vi "Facade.vi"(0 "Data In":T7, 2 "Display State In":T2, 3 "Container State":T6) -> (6 "Data Out":T7, 7 "Display State Out":T2, 8 "Action":T1)   [LabVIEW 2020, in "FSM Editor.xctl"]
uses:
  FSM Editor.xctl
  <vilib>/_xctls/Action.ctl
  <vilib>/_xctls/XControlSupport.lvlib
  Classes/FSM.Graph/FSM.Graph.lvclass
  <vilib>/Utility/cursorutil.llb/Set Cursor (Icon Pict).vi
  Drag Mode.ctl
  Classes/FSM.Edge/FSM.Edge.lvclass
  <vilib>/_xctls/Container State.ctl
  Data.vi
  State.vi
  <vilib>/Utility/miscctls.llb/LVPoint32TypeDef.ctl
  Classes/FSM.Port/FSM.Port.lvclass
  Events.ctl
  NodeAdded.ctl
  NodeSelected.ctl
  EdgeEventData.ctl
panel:
  out "picture":picture
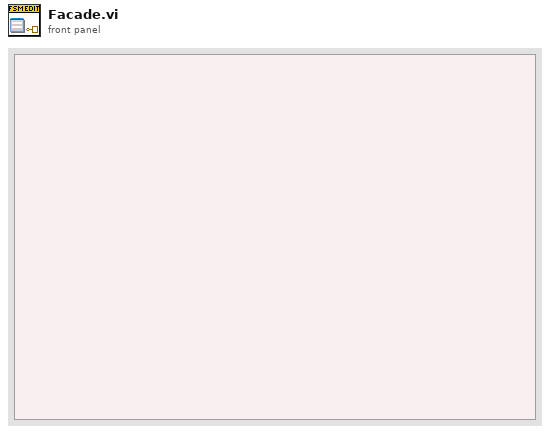
[diagram p1: front panel]
types:
  T1 = typedef "XControlSupport.lvlib/Action.ctl" = cluster{"Data Changed?":bool, "State Changed?":bool, "Action Name":string}
  T2 = typedef "FSM Editor.xctl/State.vi" = cluster{"snap":bool, "default name":string, "dragStartPoint":T3, "dragMode":T4, "gridsize":dbl, "selectRect":cluster{"left":i16, "top":i16, "right":i16, "bottom":i16}, "events":string[], "cs+/cs-":bool, "insertEdgeAt":string, "insertingEdge":bool, "activePort":refnum<class "FSM.Port.lvclass">, "sourcePort":refnum<class "FSM.Port.lvclass">, "insertionEnd":cluster{"x":i16, "y":i16}, "insertEdgeSpec":string, "nodeIndex":i32, "Events":T5, "action":string}
  T3 = typedef "LVPoint32TypeDef.ctl" = cluster{"Horizontal":i32, "Vertical":i32}
  T4 = typedef "Drag Mode.ctl" = enum16{"Off", "NodePending", "Nodes", "Pan", "Select", "EdgeInsertion", "EdgePoint", "EdgeLabel"}
  T5 = typedef "FSM Editor.xctl/Events.ctl" = cluster{"NodeAdded":refnum<user-event>, "NodeSelected":refnum<user-event>, "NodeDeleted":refnum<user-event>, "EdgeAdded":refnum<user-event>, "EdgeDeleted":refnum<user-event>, "EdgeSelected":refnum<user-event>}
  T6 = typedef "XControlSupport.lvlib/Container State.ctl" = cluster{"Indicator?":bool, "Run Mode?":bool, " Refnum":refnum<vi>}
  T7 = typedef "FSM Editor.xctl/Data.vi" = refnum<class "FSM.Graph.lvclass">
  T8 = cluster{"left":i16, "top":i16, "right":i16, "bottom":i16}
  T9 = cluster{"SourceName":string, "TargetName":string, "Accessors:Text":string, "Type":string}
  T10 = cluster{"Shift":bool, "Ctrl":bool, "Alt":bool, "Cmd":bool, "Opt":bool}
  T11 = typedef "LVBoundsTypeDef.ctl" = cluster{"Width":u32, "Height":u32}
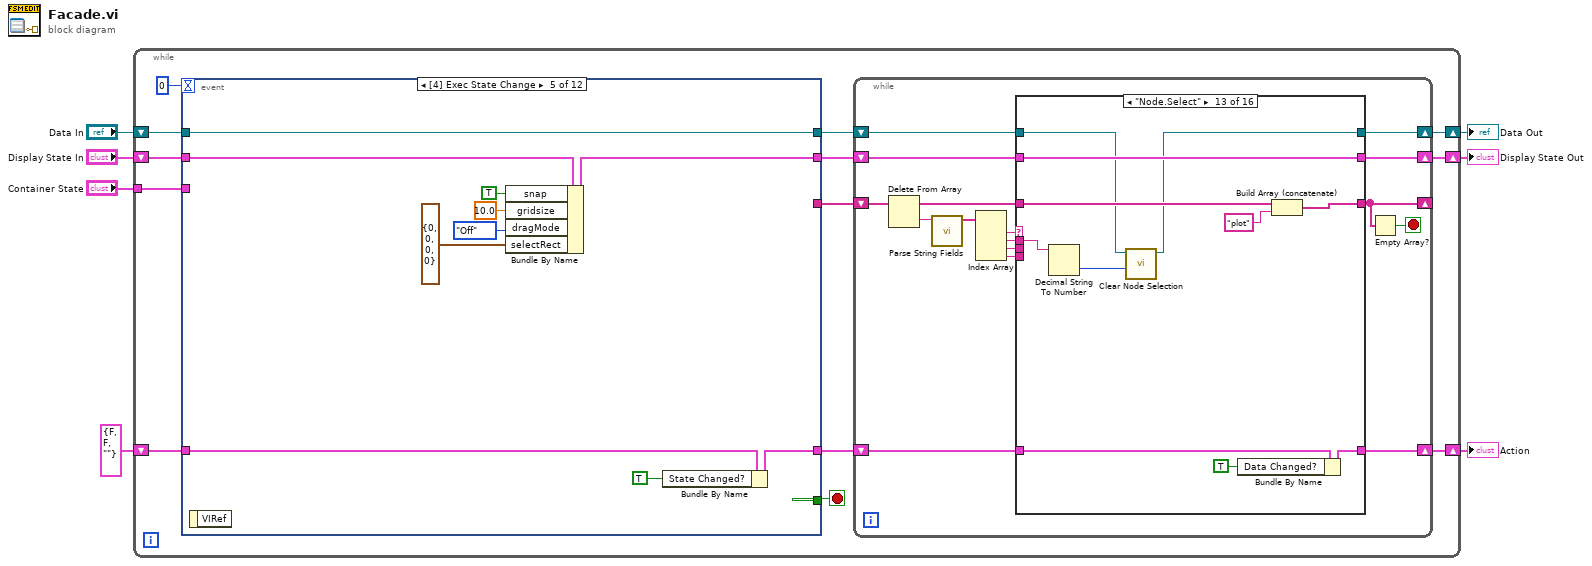
[diagram p0: block diagram]
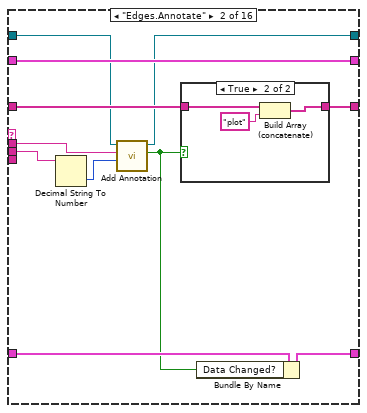
[diagram p3: hidden frame]
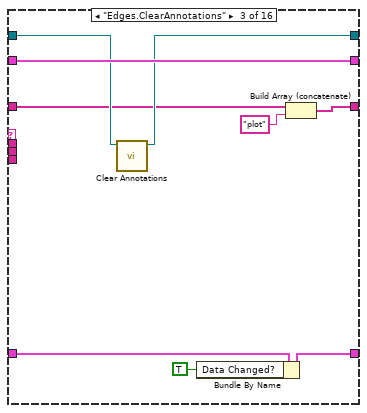
[diagram p5: hidden frame]
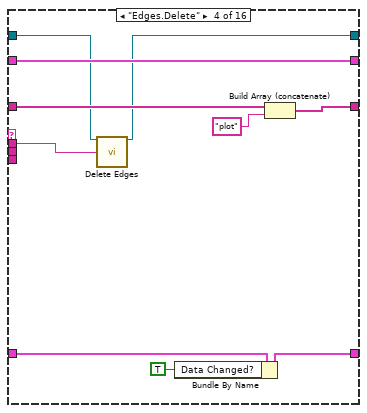
[diagram p6: hidden frame]
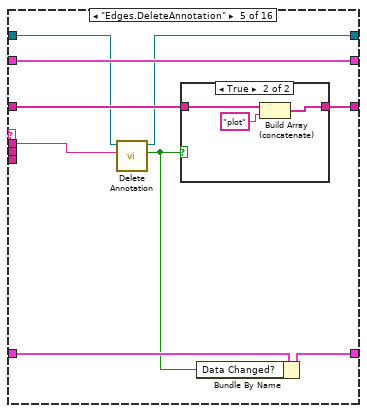
[diagram p7: hidden frame]
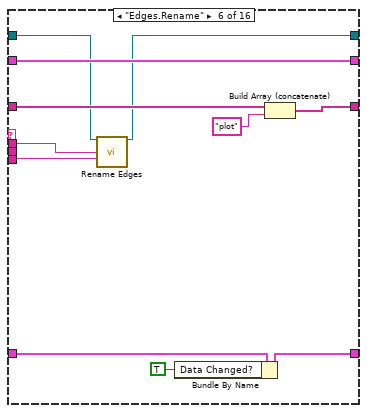
[diagram p9: hidden frame]
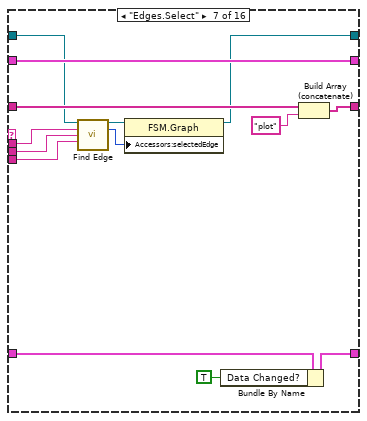
[diagram p10: hidden frame]
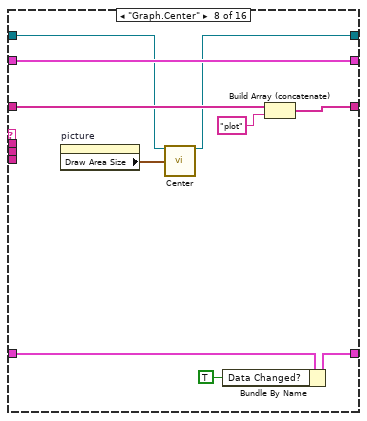
[diagram p11: hidden frame]
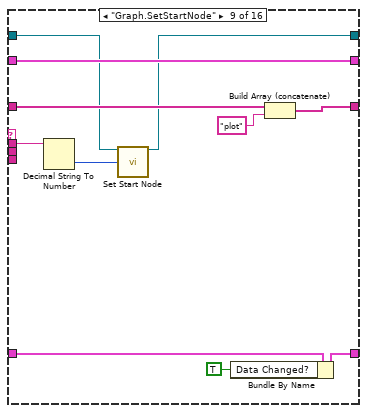
[diagram p12: hidden frame]
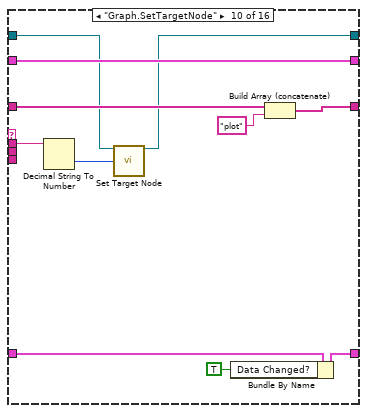
[diagram p13: hidden frame]
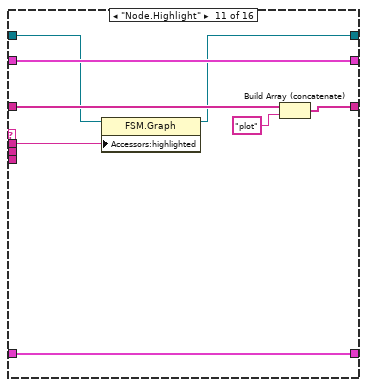
[diagram p14: hidden frame]
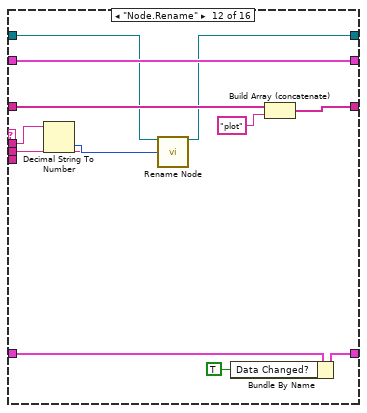
[diagram p15: hidden frame]
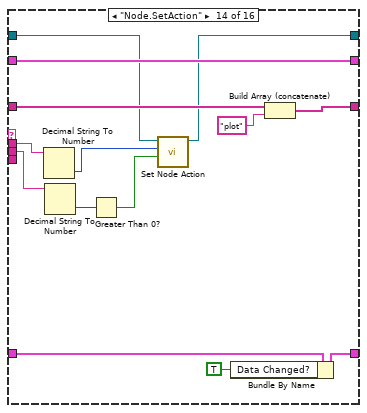
[diagram p16: hidden frame]
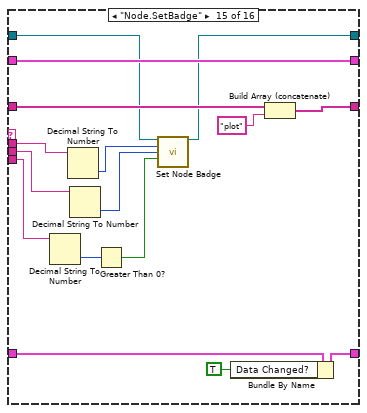
[diagram p17: hidden frame]
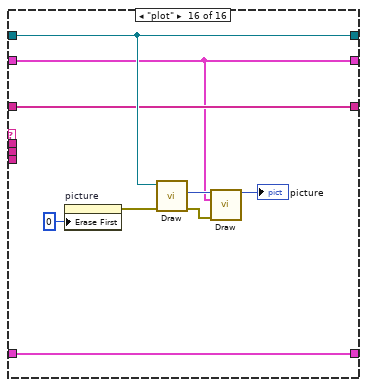
[diagram p18: hidden frame]
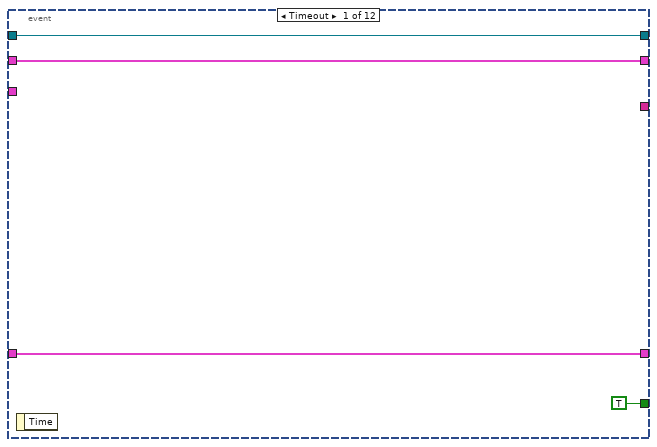
[diagram p19: hidden frame]
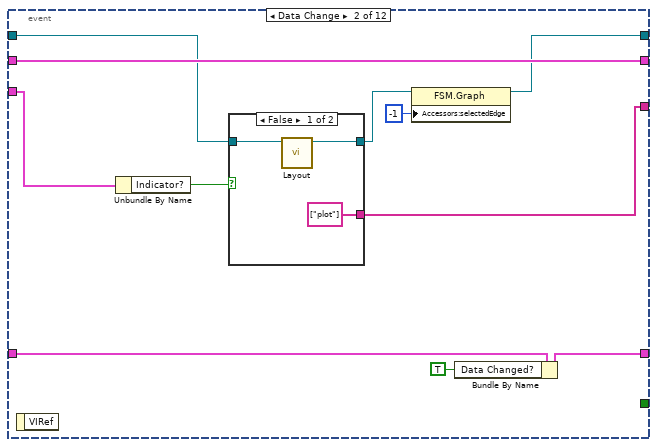
[diagram p20: hidden frame]
diagram:
  n1 = while {
    shift-right: [w10] -> w4
    shift-left: "Display State In" -> [w20]
    tunnel: "Container State" -> [w17]
    shift-right: [w8] -> w7
    shift-left: "Data In" -> [w16]
    shift-right: [w11] -> w2
    shift-left: T1 {"Data Changed?"=FALSE, "State Changed?"=FALSE, "Action Name"=""} ("Action") -> [w15]
    stop <- w19 stop-if-true
    n2 = event shown="[4] Exec State Change" {
      selector: _ -> [_ _ _ _ _ _ _ _ _ _ _ _]
      dyn-events: _ -> [_ _ _ _ _ _ _ _ _ _ _ _]
      timeout: 0 -> [_ _ _ _ _ _ _ _ _ _ _ _]
      tunnel: w20 -> [w216 w229 w241 w246 w256 w269 w273 w295 w362 w383 w399 w425]
      tunnel: [w216 w229 w238 w246 w254 w269 w276 w289 w361 w382 w398 w420] -> w13
      tunnel: [TRUE _ _ _ _ _ _ _ _ _ _ _] -> w19
      tunnel: w17 -> [_ w223 _ _ _ _ w271 w284 w357 _ w389 w416]
      tunnel: w16 -> [w215 w220 w243 w245 w247 w268 w278 w293 w363 w384 w401 w424]
      tunnel: [w215 w226 w243 w245 w247 w268 w277 w292 w364 w385 w400 w424] -> w9
      tunnel: [w217 w225 w236 w244 w253 w267 w275 w291 w358 w380 w391 w422] -> w12
      tunnel: w15 -> [w217 w228 w242 w244 w255 w267 w280 w296 w365 w386 w402 w423]
      tunnel: [_ w221 w239 _ _ _ _ w281 _ w378 w394 string[] ["plot"] ("f")] -> w14
      event Timeout {
        n3 = event-data() -> ()  [unwired: 1 in, 1 out]
      }
      event Data Change {
        n4 = event-data() -> ()  [unwired: 1 in, 1 out]
        n5 = Unbundle By Name(w223) -> ("Indicator?"=w222:bool)
        n6 = case shown="False" w222 {
          tunnel: [string[] ["plot"] string[] ["Graph.Center"]] -> w221
          tunnel: w220 -> [w231 w233]
          tunnel: [w230 w233] -> w219
          frame False {
            n7 = call "Layout.vi"("FSM in"=w231) -> ("FSM out"=w230:T7)  [unwired: 9 in, 1 out]
          }
          frame True {
          }
        }
        n8 = property class="FSM.Graph"(reference=w219, "Accessors:selectedEdge"=-1 ("selectedEdge")) -> (reference out=w226:T7)  [unwired: 1 in, 1 out]
        n9 = Bundle By Name(cluster=w228, "Data Changed?"=TRUE) -> (w225:T1)
      }
      event Display State Change {
        n10 = event-data() -> ()  [unwired: 1 in, 1 out]
        n11 = Unbundle By Name(w241) -> ("action"=w240:string)
        n12 = Bundle By Name(cluster=w242, "State Changed?"=TRUE) -> (w236:T1)
        n13 = Bundle By Name(cluster=w241, "action"="") -> (w238:T2)
        n14 = Build Array(w240) -> (w239:string[])
      }
      event Direction Change {
        n15 = event-data() -> ()  [unwired: 1 in, 1 out]
      }
      event Exec State Change {
        n16 = event-data() -> ()  [unwired: 1 in, 1 out]
        n17 = Bundle By Name(cluster=w256, "snap"=TRUE, "gridsize"=10.0, "dragMode"=Drag_Mode."Off", "selectRect"=T8 {"left"=0, "top"=0, "right"=0, "bottom"=0}) -> (w254:T2)
        n18 = Bundle By Name(cluster=w255, "State Changed?"=TRUE) -> (w253:T1)
      }
      event Panel Resize {
        w260 = i16 10
        n19 = event-data() -> ("NewBnds.Right"=w266:i16, "NewBnds.Left"=w265:i16, "NewBnds.Bottom"=w264:i16, "NewBnds.Top"=w263:i16)  [unwired: 1 in]
        n20 = Subtract(x=w266, y=w265) -> (x-y=w262:i16)
        n21 = Subtract(x=w264, y=w263) -> (x-y=w261:i16)
        n22 = Add(x=w262, y=w260) -> (x+y=w259:i16)
        n23 = Add(x=w261, y=w260) -> (x+y=w258:i16)
        n24 = Bundle(w259, w258) -> (w257:cluster{i16, i16})  [unwired: 1 in]
        n25 = property on="picture" class="Pict"("Draw Area Size"=w257) -> ()  [unwired: 2 in, 2 out]
      }
      event "picture": Shortcut Menu Activation? {
        n26 = event-data() -> ("MenuRef"=w272:refnum<k9>, "Coords"=w279:T3)  [unwired: 1 in]
        n27 = Unbundle By Name(w271) -> ("Indicator?"=w270:bool)
        n28 = call "Build Context Menu.vi"("FSM.Graph in"=w278, "Display State In in"=w273, "MenuRef"=w272, "Coords"=w279) -> ("FSM.Graph out"=w277:T7, "Display State In out"=w276:T2)  [unwired: 10 in]
        n29 = Bundle By Name(cluster=w280, "State Changed?"=TRUE) -> (w275:T1)
        n30 = event-data("Discard?"=w270) -> ()  [unwired: 1 in, 1 out]
      }
      event "picture": Shortcut Menu Selection (User) {
        w286 = TRUE ("Data Changed?")
        n31 = event-data() -> ("CtlRef"=w285:refnum<vi>, "Coords"=w294:T3, "ItemPath"=w290:string, "ItemTag"=w282:string)  [unwired: 1 in]
        n32 = Unbundle By Name(w284) -> ("Refnum"=w283:refnum<vi>)
        n33 = Search/Split String(string=w282, search string/char (-)=":") -> (substring before match=w287:string)  [unwired: 1 in, 2 out]
        n34 = case shown="\"cmDeleteSelected\"" w287 {
          tunnel: w295 -> [w297 w303 w309 w319 w322 w326 w339 w344 w348]
          tunnel: w294 -> [_ w305 _ _ _ _ _ w341 _]
          tunnel: w293 -> [w298 w307 w310 w318 w321 w329 w338 w343 w347]
          tunnel: [w298 w306 w315 w317 w321 w328 w337 w342 w346] -> w292
          tunnel: [w297 w303 w309 w319 w322 w326 w336 w344 w348] -> w289
          tunnel: w290 -> [_ _ _ _ _ _ _ _ _]
          tunnel: w285 -> [_ _ _ _ _ _ _ _ _]
          tunnel: w283 -> [_ _ _ _ _ _ w333 _ _]
          tunnel: w282 -> [_ _ _ _ _ _ w331 _ _]
          tunnel: [_ string[] ["plot"] string[] ["plot"] string[] ["plot"] string[] ["Graph.Center"] string[] ["plot"] string[] ["plot"] string[] ["plot"] string[] ["plot"]] -> w281
          frame "", Default {
          }
          frame "cmInsertNode" {
            n35 = Unbundle By Name(w303) -> ("default name"=w308:string)
            n36 = call "Snap To Grid.vi"("Display State In"=w303, "Point In"=w305) -> ("Point Out"=w304:cluster{"Horizontal":dbl, "Vertical":dbl})  [unwired: 13 in]
            n37 = Unbundle By Name(w303) -> ("Events.NodeAdded"=w302:refnum<user-event>)
            n38 = call "AddNodeAutoName.vi"("Default Node Name"=w308, "point"=w304, "FSM in"=w307) -> ("Name"=w301:string, "FSM out"=w306:T7)  [unwired: 6 in, 1 out]
            n39 = Bundle("Name"=w301) -> (w300:cluster{"Name":string})  [unwired: 1 in]
            n40 = Generate User Event(user event=w302, event data cluster=w300) -> ()  [unwired: 2 in, 2 out]
          }
          frame "cmDeleteSelected" {
            n41 = Unbundle By Name(w309) -> ("Events.NodeDeleted"=w313:refnum<user-event>)
            n42 = property class="FSM.Graph"(reference=w310) -> ("Accessors:selectedNodes"=w312:i32[])  [unwired: 1 in, 2 out]
            n43 = call "Delete Selected Nodes.vi"("FSM in"=w310) -> ("FSM out"=w315:T7)  [unwired: 9 in, 1 out]
            n44 = Bundle("Accessors:selectedNodes"=w312) -> (w311:cluster{"Accessors:selectedNodes":i32[]})  [unwired: 1 in]
            n45 = Generate User Event(user event=w313, event data cluster=w311) -> ()  [unwired: 2 in, 2 out]
          }
          frame "cmAnnotate" {
            n46 = call "Toggle Selected Edge Annotation Shown.vi"("FSM in"=w318) -> ("FSM out"=w317:T7)  [unwired: 9 in, 1 out]
          }
          frame "cmCenter" {
          }
          frame "cmDeleteSelectedEdge" {
            n47 = call "Delete Edge.vi"("FSM.Graph In"=w329) -> ("FSM.Graph Out"=w328:T7, "Deleted Edge"=w327:refnum<class "FSM.Edge.lvclass">)  [unwired: 13 in]
            n48 = call "Get Event Data.vi"("FSM.Edge in"=w327) -> ("Event Data"=w324:T9)  [unwired: 8 in, 2 out]
            n49 = Unbundle By Name(w326) -> ("Events.EdgeDeleted"=w325:refnum<user-event>)
            n50 = Generate User Event(user event=w325, event data cluster=w324) -> ()  [unwired: 2 in, 2 out]
          }
          frame "cmInsert", "cmInsertAny", "cmInsertCS+", "cmInsertCS-" {
            n51 = property class="Ctl"(reference=w333) -> ("OwningVI"=w332:refnum<vi>)  [unwired: 1 in, 2 out]
            n52 = call "Clear Node Selection.vi"("FSM in"=w338) -> ("FSM out"=w337:T7)  [unwired: 9 in, 1 out]
            n53 = call-poly <vilib>:"Set Cursor.vi"("VI reference (current VI)"=w332, "icon"=u16 4) -> ()  [unwired: 8 in, 2 out]
            n54 = Bundle By Name(cluster=w339, "insertingEdge"=TRUE, "insertEdgeSpec"=w331) -> (w336:T2)
          }
          frame "cmInsertControlPoint" {
            n55 = call "Insert Edge Point.vi"("FSM.Graph In"=w343, "Location"=w341) -> ("FSM.Graph Out"=w342:T7)  [unwired: 13 in]
          }
          frame "cmDeleteControlPoint" {
            n56 = call "Delete Edge Point.vi"("FSM.Graph In"=w347) -> ("FSM.Graph Out"=w346:T7)  [unwired: 14 in]
          }
        }
        n57 = Bundle By Name(cluster=w296, "Data Changed?"=w286, "State Changed?"=w286) -> (w291:T1)
      }
      event "picture": Mouse Down {
        w355 = TRUE ("State Changed?")
        n58 = event-data() -> ("Coords"=w360:T3, "PlatMods"=w359:T10, "Button"=w354:u16)  [unwired: 1 in]
        n59 = Unbundle By Name(w357) -> ("Refnum"=w356:refnum<vi>, "Indicator?"=w352:bool)
        n60 = Not(x=w352) -> (.not. x?=w351:bool)
        n61 = Equal?(x=w354, y=u16 1) -> (x = y?=w350:bool)
        n62 = And(x=w351, y=w350) -> (x .and. y?=w349:bool)
        n63 = case shown="True" w349 {
          tunnel: [w367 w374] -> w364
          tunnel: w363 -> [w367 w373]
          tunnel: w362 -> [w366 w372]
          tunnel: [w366 w371] -> w361
          tunnel: w360 -> [_ w370]
          tunnel: w359 -> [_ w369]
          tunnel: w356 -> [_ w368]
          frame False {
          }
          frame True {
            n64 = call "Process Mouse Down.vi"("FSM.Graph in"=w373, "Display State In"=w372, "Coords"=w370, "PlatMods"=w369, "Editor Ref"=w368) -> ("FSM.Graph out"=w374:T7, "Display State Out"=w371:T2)  [unwired: 9 in]
          }
        }
        n65 = Bundle By Name(cluster=w365, "Data Changed?"=w355, "State Changed?"=w355) -> (w358:T1)
      }
      event "picture": Mouse Move {
        w379 = TRUE ("State Changed?")
        n66 = event-data() -> ("Coords"=w381:T3)  [unwired: 1 in]
        n67 = call "Process Mouse Move.vi"("FSM.Graph in"=w384, "Display State In"=w383, "Coords"=w381) -> ("FSM.Graph out"=w385:T7, "Display State Out"=w382:T2, "Refresh"=w377:bool)  [unwired: 10 in]
        n68 = Select(t=string[] ["plot"], s=w377, f=string[] []) -> (s? t:f=w378:string[])
        n69 = Bundle By Name(cluster=w386, "Data Changed?"=w379, "State Changed?"=w379) -> (w380:T1)
      }
      event "picture": Mouse Up {
        w390 = TRUE ("State Changed?")
        n70 = event-data() -> ("Coords"=w397:T3, "PlatMods"=w392:T10)  [unwired: 1 in]
        n71 = Unbundle By Name(w389) -> ("Indicator?"=w387:bool, "Refnum"=w388:refnum<vi>)
        n72 = case shown="False" w387 {
          tunnel: w401 -> [w410 w412]
          tunnel: [w409 w412] -> w400
          tunnel: w399 -> [w408 w411]
          tunnel: [w407 w411] -> w398
          tunnel: w397 -> [w406 _]
          tunnel: [w405 _] -> w393
          tunnel: w392 -> [w404 _]
          tunnel: w388 -> [w403 _]
          frame False {
            n73 = call "Process Mouse Up.vi"("FSM.Graph in"=w410, "Display State In"=w408, "Coords"=w406, "PlatMods"=w404, "Editor Ref"=w403) -> ("FSM.Graph out"=w409:T7, "Display State Out"=w407:T2, "Refresh"=w405:bool)  [unwired: 8 in]
          }
          frame True {
          }
        }
        n74 = Bundle By Name(cluster=w402, "State Changed?"=w390, "Data Changed?"=w390) -> (w391:T1)
        n75 = Select(t=string[] ["plot"], s=w393, f=string[] []) -> (s? t:f=w394:string[])
      }
      event "picture": Mouse Leave {
        n76 = event-data() -> ()  [unwired: 1 in, 1 out]
        n77 = Unbundle By Name(w416) -> ("Refnum"=w415:refnum<vi>)
        n78 = property class="Ctl"(reference=w415) -> ("OwningVI"=w418:refnum<vi>)  [unwired: 1 in, 2 out]
        n79 = call-poly <vilib>:"Set Cursor.vi"("VI reference (current VI)"=w418, "icon"=u16 0) -> ()  [unwired: 8 in, 2 out]
        n80 = Bundle By Name(cluster=w425, "dragMode"=Drag_Mode."Off", "insertingEdge"=FALSE) -> (w420:T2)
        n81 = Bundle By Name(cluster=w423, "State Changed?"=TRUE ("Data Changed?")) -> (w422:T1)
      }
    }
    n82 = while {
      shift-right: [w34] -> _
      shift-left: w14 -> [w36]
      shift-right: [w30] -> w11
      shift-left: w12 -> [w31]
      shift-right: [w29] -> w10
      shift-left: w13 -> [w32]
      shift-right: [w27] -> w8
      shift-left: w9 -> [w28]
      stop <- w33 stop-if-true
      n83 = Delete From Array(array=w36) -> (deleted portion=w26:string, array with subset deleted=w35:string[])  [unwired: 2 in]
      n84 = call "Parse String Fields.vi"("String"=w26) -> ("Fields"=w25:string[])  [unwired: 9 in, 1 out]
      n85 = Index Array(array=w25) -> (element #1=w24:string, element #2=w23:string, element #3=w22:string, element #4=w21:string)  [unwired: 4 in]
      n86 = case shown="\"Node.Select\"" w24 {
        tunnel: w35 -> [w40 w51 w60 w74 w83 w98 w112 w122 w133 w144 w149 w164 w175 w189 w205 w210]
        tunnel: [w40 w43 w57 w68 w77 w91 w109 w119 w130 w141 w148 w159 w172 w184 w200 w210] -> w34
        tunnel: w32 -> [w38 w49 w63 w72 w81 w96 w110 w120 w131 w142 w151 w162 w173 w187 w203 w206]
        tunnel: w31 -> [w39 w50 w64 w73 w82 w97 w111 w121 w132 w143 w152 w163 w174 w188 w204 w212]
        tunnel: [w39 w42 w59 w66 w76 w89 w107 w117 w128 w139 w152 w157 w170 w182 w198 w212] -> w30
        tunnel: [w38 w49 w63 w72 w81 w96 w110 w120 w131 w142 w151 w162 w173 w187 w203 w206] -> w29
        tunnel: w28 -> [w37 w48 w62 w70 w80 w93 w105 w115 w125 w136 w147 w161 w167 w186 w202 w211]
        tunnel: [w37 w47 w61 w69 w79 w92 w99 w113 w124 w135 w146 w160 w165 w185 w201 w211] -> w27
        tunnel: w23 -> [_ w46 _ w71 w78 w95 w104 _ w126 w137 w145 w155 w168 w180 w196 _]
        tunnel: w22 -> [_ w45 _ _ _ w94 w103 _ _ _ _ w153 _ w178 w191 _]
        tunnel: w21 -> [_ _ _ _ _ _ w102 _ _ _ _ _ _ _ w193 _]
        frame "", Default {
        }
        frame "Edges.Annotate" {
          n87 = Decimal String To Number(string=w45) -> (number=w44:i32)  [unwired: 2 in, 1 out]
          n88 = call "Add Annotation.vi"("Style"=w44, "Name"=w46, "FSM in"=w48) -> ("Changed?"=w41:bool, "FSM out"=w47:T7)  [unwired: 6 in, 1 out]
          n89 = case shown="True" w41 {
            tunnel: w51 -> [w52 w55]
            tunnel: [w52 w54] -> w43
            frame False {
            }
            frame True {
              n90 = Build Array (concatenate)(w55, "plot") -> (w54:string[])
            }
          }
          n91 = Bundle By Name(cluster=w50, "Data Changed?"=w41) -> (w42:T1)
        }
        frame "Edges.ClearAnnotations" {
          n92 = call "Clear Annotations.vi"("FSM in"=w62) -> ("FSM out"=w61:T7)  [unwired: 9 in, 1 out]
          n93 = Bundle By Name(cluster=w64, "Data Changed?"=TRUE) -> (w59:T1)
          n94 = Build Array (concatenate)(w60, "plot") -> (w57:string[])
        }
        frame "Edges.Delete" {
          n95 = call "Delete Edges.vi"("FSM.Graph In"=w70, "Name"=w71) -> ("FSM.Graph Out"=w69:T7)  [unwired: 13 in]
          n96 = Bundle By Name(cluster=w73, "Data Changed?"=TRUE) -> (w66:T1)
          n97 = Build Array (concatenate)(w74, "plot") -> (w68:string[])
        }
        frame "Edges.DeleteAnnotation" {
          n98 = call "Delete Annotation.vi"("Name"=w78, "FSM in"=w80) -> ("Changed?"=w75:bool, "FSM out"=w79:T7)  [unwired: 7 in, 1 out]
          n99 = case shown="True" w75 {
            tunnel: w83 -> [w84 w87]
            tunnel: [w84 w86] -> w77
            frame False {
            }
            frame True {
              n100 = Build Array (concatenate)(w87, "plot") -> (w86:string[])
            }
          }
          n101 = Bundle By Name(cluster=w82, "Data Changed?"=w75) -> (w76:T1)
        }
        frame "Edges.Rename" {
          n102 = call "Rename Edges.vi"("FSM.Graph In"=w93, "Old Name"=w95, "New Name"=w94) -> ("FSM.Graph Out"=w92:T7)  [unwired: 12 in]
          n103 = Bundle By Name(cluster=w97, "Data Changed?"=TRUE) -> (w89:T1)
          n104 = Build Array (concatenate)(w98, "plot") -> (w91:string[])
        }
        frame "Edges.Select" {
          n105 = call "Find Edge.vi"("FSM in"=w105, "From"=w104, "To"=w103, "Type"=w102) -> ("FSM thru"=w101:T7, "Edge Index"=w100:i32)  [unwired: 9 in, 1 out]
          n106 = property class="FSM.Graph"(reference=w101, "Accessors:selectedEdge"=w100) -> (reference out=w99:T7)  [unwired: 1 in, 1 out]
          n107 = Bundle By Name(cluster=w111, "Data Changed?"=TRUE) -> (w107:T1)
          n108 = Build Array (concatenate)(w112, "plot") -> (w109:string[])
        }
        frame "Graph.Center" {
          n109 = property on="picture" class="Pict"() -> ("Draw Area Size"=w114:T11)  [unwired: 2 in, 2 out]
          n110 = call "Center.vi"("FSM.Graph In"=w115, "Draw Area Size"=w114) -> ("FSM.Graph Out"=w113:T7)  [unwired: 13 in]
          n111 = Bundle By Name(cluster=w121, "Data Changed?"=TRUE) -> (w117:T1)
          n112 = Build Array (concatenate)(w122, "plot") -> (w119:string[])
        }
        frame "Graph.SetStartNode" {
          n113 = Decimal String To Number(string=w126) -> (number=w123:i32)  [unwired: 2 in, 1 out]
          n114 = call "Set Start Node.vi"("FSM.Graph In"=w125, "Index"=w123) -> ("FSM.Graph Out"=w124:T7)  [unwired: 13 in]
          n115 = Bundle By Name(cluster=w132, "Data Changed?"=TRUE) -> (w128:T1)
          n116 = Build Array (concatenate)(w133, "plot") -> (w130:string[])
        }
        frame "Graph.SetTargetNode" {
          n117 = Decimal String To Number(string=w137) -> (number=w134:i32)  [unwired: 2 in, 1 out]
          n118 = call "Set Target Node.vi"("FSM.Graph In"=w136, "Index"=w134) -> ("FSM.Graph Out"=w135:T7)  [unwired: 13 in]
          n119 = Bundle By Name(cluster=w143, "Data Changed?"=TRUE) -> (w139:T1)
          n120 = Build Array (concatenate)(w144, "plot") -> (w141:string[])
        }
        frame "Node.Highlight" {
          n121 = property class="FSM.Graph"(reference=w147, "Accessors:highlighted"=w145) -> (reference out=w146:T7)  [unwired: 1 in, 1 out]
          n122 = Build Array (concatenate)(w149, "plot") -> (w148:string[])
        }
        frame "Node.Rename" {
          n123 = Decimal String To Number(string=w155) -> (number=w154:i32)  [unwired: 2 in, 1 out]
          n124 = call "Rename Node.vi"("FSM.Graph In"=w161, "Index"=w154, "New name"=w153) -> ("FSM.Graph Out"=w160:T7)  [unwired: 12 in]
          n125 = Bundle By Name(cluster=w163, "Data Changed?"=TRUE) -> (w157:T1)
          n126 = Build Array (concatenate)(w164, "plot") -> (w159:string[])
        }
        frame "Node.Select" {
          n127 = Decimal String To Number(string=w168) -> (number=w166:i32)  [unwired: 2 in, 1 out]
          n128 = call "Clear Node Selection.vi"("New selection"=w166, "FSM in"=w167) -> ("FSM out"=w165:T7)  [unwired: 8 in, 1 out]
          n129 = Bundle By Name(cluster=w174, "Data Changed?"=TRUE) -> (w170:T1)
          n130 = Build Array (concatenate)(w175, "plot") -> (w172:string[])
        }
        frame "Node.SetAction" {
          n131 = Decimal String To Number(string=w180) -> (number=w179:i32)  [unwired: 2 in, 1 out]
          n132 = Decimal String To Number(string=w178) -> (number=w177:i32)  [unwired: 2 in, 1 out]
          n133 = Greater Than 0?(x=w177) -> (x > 0?=w176:bool)
          n134 = call "Set Node Action.vi"("action-only"=w176, "nodeIndex"=w179, "FSM in"=w186) -> ("FSM out"=w185:T7)  [unwired: 7 in, 1 out]
          n135 = Bundle By Name(cluster=w188, "Data Changed?"=TRUE) -> (w182:T1)
          n136 = Build Array (concatenate)(w189, "plot") -> (w184:string[])
        }
        frame "Node.SetBadge" {
          n137 = Decimal String To Number(string=w193) -> (number=w194:i32)  [unwired: 2 in, 1 out]
          n138 = Decimal String To Number(string=w196) -> (number=w195:i32)  [unwired: 2 in, 1 out]
          n139 = Decimal String To Number(string=w191) -> (number=w190:i32)  [unwired: 2 in, 1 out]
          n140 = Greater Than 0?(x=w194) -> (x > 0?=w192:bool)
          n141 = call "Set Node Badge.vi"("FSM in"=w202, "nodeIndex"=w195, "Badge"=w190, "visible"=w192) -> ("FSM out"=w201:T7)  [unwired: 10 in, 1 out]
          n142 = Bundle By Name(cluster=w204, "Data Changed?"=TRUE) -> (w198:T1)
          n143 = Build Array (concatenate)(w205, "plot") -> (w200:string[])
        }
        frame "plot" {
          n144 = property on="picture" class="Pict"("Erase First"=u8 0) -> (error out=w213:errorcluster)  [unwired: 2 in, 1 out]
          n145 = call "Draw.vi"("error in (no error)"=w213, "FSM in"=w211) -> ("error out"=w209:errorcluster, "picture out"=w208:picture)  [unwired: 7 in, 1 out]
          n146 = call "Draw.vi"("picture in"=w208, "Display State"=w206, "error in (no error)"=w209) -> ("picture out"=→"picture":picture)  [unwired: 12 in]
        }
      }
      n147 = Empty Array?(array=w34) -> (empty?=w33:bool)
    }
  }
  "Display State Out" <- w4
  "Data Out" <- w7
  "Action" <- w2
